vi "TestLeakage.vi"(4 "Voltage Level DxSupply":dbl, 5 "Voltage Level DxBoot0":dbl, 6 "Current Limit DxSupply":dbl, 7 "Current Limit  DxBoot0":dbl, 8 "error in (no error)":errorcluster, 9 "DxSupply":string="0", 10 "DxBoot0":string="0", 11 "IVI Refnum in":refnum<k15>) -> (0 "error out":errorcluster, 1 "Idd Average DxSupply":dbl format="%0.2f", 2 "Idd Average DxBoot0":dbl format="%0.2f")   [LabVIEW 2018]
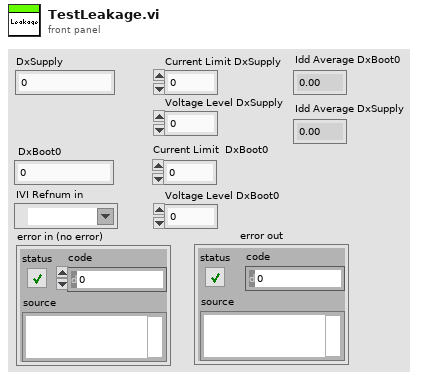
[diagram p1: front panel]
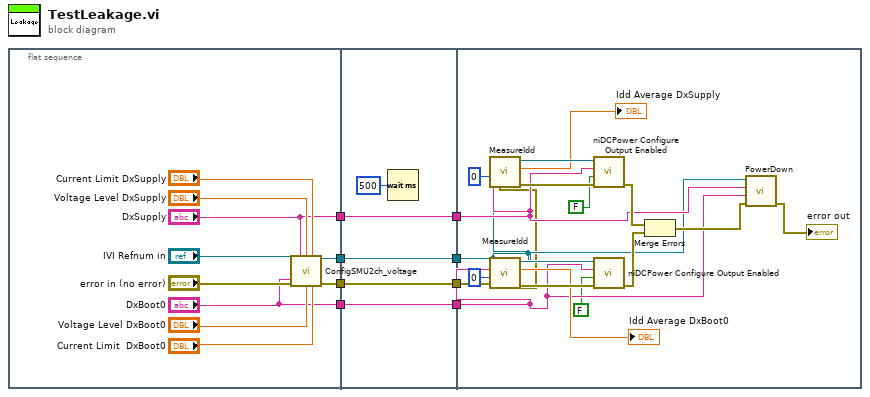
[diagram p0: block diagram]
diagram:
  n1 = flat-sequence {
    tunnel: [w12] -> w8
    tunnel: [w11] -> w7
    tunnel: ["DxBoot0"] -> w6
    tunnel: ["DxSupply"] -> w5
    tunnel: w8 -> [w23]
    tunnel: w7 -> [w22]
    tunnel: w6 -> [w21]
    tunnel: w5 -> [w20]
    tunnel: [w23] -> w4
    tunnel: [w22] -> w3
    tunnel: [w21] -> w2
    tunnel: [w20] -> w1
    tunnel: w4 -> [w28]
    tunnel: w3 -> [w29]
    tunnel: w2 -> [w31]
    tunnel: w1 -> [w30]
    frame #0 {
      n2 = call "ConfigSMU2ch_voltage.vi"("IVI Refnum in"="IVI Refnum in", "Channel DxSupply"="DxSupply", "Voltage Level DxSupply"="Voltage Level DxSupply", "Current Limit DxSupply"="Current Limit DxSupply", "error in (no error)"="error in (no error)", "Channel DxBoot0"="DxBoot0", "Voltage Level DxBoot0"="Voltage Level DxBoot0", "Current Limit DxBoot0"="Current Limit  DxBoot0") -> ("IVI Refnum out"=w11:refnum<k15>, "error out"=w12:errorcluster)  [unwired: 6 in]
    }
    frame #1 {
      n3 = Wait (ms)(milliseconds to wait=u32 500) -> ()  [unwired: 1 out]
    }
    frame #2 {
      n4 = call "MeasureIdd.vi"("error in (no error)"=w28, "Deep Sleep Time"=u32 0, "channel name"=w30, "instrument handle"=w29) -> ("error out"=w37:errorcluster, "Idd Average"=→"Idd Average DxSupply":dbl, "instrument handle out"=w36:refnum<k15>)  [unwired: 5 in]
      n5 = call "MeasureIdd.vi"("error in (no error)"=w28, "Deep Sleep Time"=u32 0, "channel name"=w31, "instrument handle"=w29) -> ("error out"=w34:errorcluster, "Idd Average"=→"Idd Average DxBoot0":dbl, "instrument handle out"=w33:refnum<k15>)  [unwired: 5 in]
      n6 = call <instrlib>:"niDCPower Configure Output Enabled.vi"("error in (no error)"=w37, "output enabled"=FALSE, "channel name"=w30, "instrument handle"=w36) -> ("error out"=w39:errorcluster)  [unwired: 7 out]
      n7 = call <instrlib>:"niDCPower Configure Output Enabled.vi"("error in (no error)"=w34, "output enabled"=FALSE, "channel name"=w31, "instrument handle"=w33) -> ("error out"=w38:errorcluster)  [unwired: 7 out]
      n8 = Merge Errors(w39, w38) -> (w40:errorcluster)
      n9 = call "PowerDown.vi"("error in (no error)"=w40, "DxBoot0"=w31, "DxSupply"=w30, "SMU handle in"=w29) -> ("error out"=→"error out":errorcluster)  [unwired: 6 in, 1 out]
    }
  }
